vi "Ctr_FindRef.vi"(8 "error in (no error)":errorcluster caption="error in", 10 "control name":string="panel0", 11 "vi*(本VI)":refnum<vi>) -> (0 "error out":errorcluster, 2 "ctrl*":refnum<vi>, 3 "vi* out":refnum<vi>)   [LabVIEW 2016]
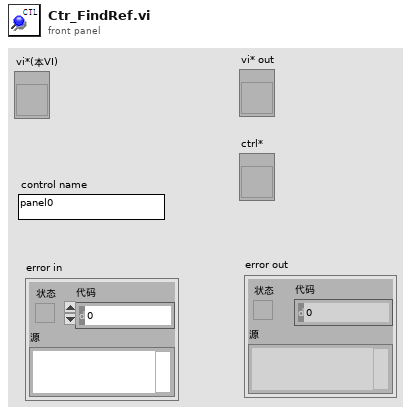
[diagram p1: front panel]
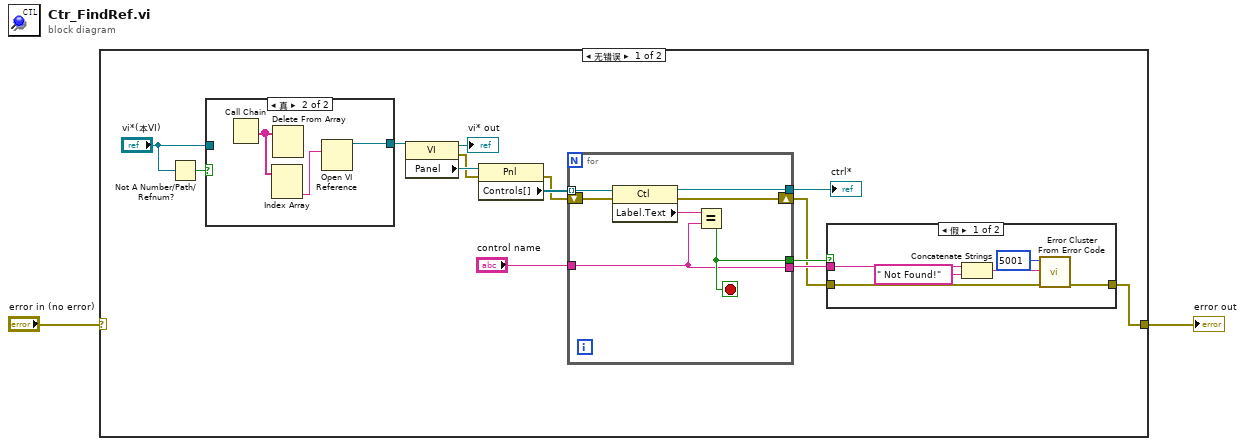
[diagram p0: block diagram]
diagram:
  n1 = case shown="无错误" "error in (no error)" {
    selector: "error in (no error)" -> [_ w35]
    tunnel: [w9 w35] -> w1
    frame No Error {
      n2 = Not A Number/Path/Refnum?(number/path/refnum="vi*(本VI)") -> (NaN/Path/Refnum?=w4:bool)
      n3 = case shown="真" w4 {
        tunnel: [w17 w20] -> w5
        tunnel: "vi*(本VI)" -> [w17 _]
        frame False {
        }
        frame True {
          n4 = Call Chain() -> (call chain=w19:string[])
          n5 = Index Array(array=w19) -> (element #2=w18:string)  [unwired: 2 in, 1 out]
          n6 = Delete From Array(array=w19) -> ()  [unwired: 2 in, 2 out]
          n7 = Open VI Reference(vi path=w18) -> (vi reference=w20:refnum<vi>)  [unwired: 5 in, 1 out]
        }
      }
      n8 = property class="VI"(reference=w5) -> (reference out=→"vi* out":refnum<vi>, error out=w11:errorcluster, "Panel"=w16:refnum<vi>)  [unwired: 1 in]
      n9 = property class="Pnl"(reference=w16, error in=w11) -> (error out=w10:errorcluster, "Controls[]"=w14:refnum<vi>[])  [unwired: 1 out]
      n10 = for {
        tunnel: w14 -> [w34] mode=indexing
        tunnel: [w32] -> w15
        tunnel: [w31] -> w12
        tunnel: [w28] -> w13
        shift-right: [w29] -> w8
        shift-left: w10 -> [w30]
        tunnel: "control name" -> [w28]
        stop <- w31 stop-if-true
        n11 = property class="Ctl"(reference=w34, error in=w30) -> (reference out=w32:refnum<vi>, error out=w29:errorcluster, "Label.Text"=w33:string)
        n12 = Equal?(x=w33, y=w28) -> (x = y?=w31:bool)
      }
      "ctrl*" <- w15
      n13 = case shown="假" w12 {
        tunnel: w13 -> [w26 _]
        tunnel: [w22 w27] -> w9
        tunnel: w8 -> [w21 w27]
        frame False {
          n14 = Concatenate Strings(w26, " Not Found!" ("字符串")) -> (w24:string)
          n15 = call <vilib>:"Error Cluster From Error Code.vi"("error in (no error)"=w21, "error message (\"\")"=w24, "error code (0)"=5001) -> ("error out"=w22:errorcluster)  [unwired: 6 in]
        }
        frame True {
        }
      }
    }
    frame Error {
    }
  }
  "error out" <- w1
